vi "HW_6p1_Task1_doanbs.vi"() -> ()   [LabVIEW 2016]
uses:
  <vilib>/express/express arith-compare/Formula/XNode/ExpressFormulaBlockNode.xnode
panel:
  out "Final Time":dbl
  out "T(t), Final Object Temp":dbl
  in  "k, Heat Transfer Coefficient":dbl
  in  "To, Initial Object Temp":dbl
  in  "Ts, Surrounding Temp":dbl
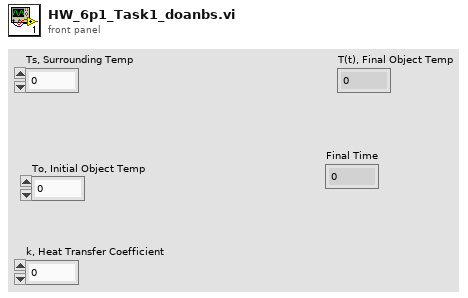
[diagram p1: front panel]
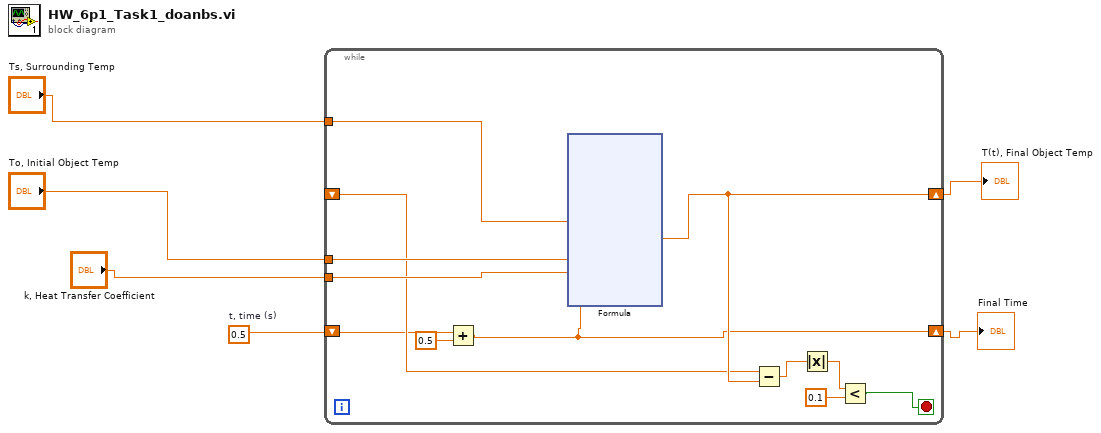
[diagram p0: block diagram]
diagram:
  w2 = 0.5  # t, time (s)
  n1 = while {
    tunnel: "k, Heat Transfer Coefficient" -> [w18]
    tunnel: "To, Initial Object Temp" -> [w17]
    tunnel: "Ts, Surrounding Temp" -> [w16]
    shift-right: [w15] -> w3
    shift-left: _ -> [w14]
    shift-right: [w9] -> w1
    shift-left: w2 -> [w10]
    stop <- w12 stop-if-true
    n2 = Add(x=w10, y=0.5) -> (x+y=w9:dbl)
    n3 = xnode "Formula"("Ts"=w16, "To"=w17, "k"=w18, "t"=w9) -> ("Result"=w15:dbl)  [unwired: 1 in, 1 out]
    n4 = Subtract(x=w14, y=w15) -> (x-y=w8:dbl)
    n5 = Absolute Value(x=w8) -> (abs(x)=w7:dbl)
    n6 = Less?(x=w7, y=0.1) -> (x < y?=w12:bool)
  }
  "T(t), Final Object Temp" <- w3
  "Final Time" <- w1
